vi "ep_Simulate.vi"(0 "signal definition":T2(array[cluster])=[{"Array"=[{"level (%)"=100.0, "phase (°)"=0.0, "harm."=1.0}, {"level (%)"=3.0, "phase (°)"=30.0, "harm."=3.0}]}, {"Array"=[{"level (%)"=100.0, "phase (°)"=-120.0, "harm."=1.0}, {"level (%)"=4.0, "phase (°)"=80.0, "harm."=7.0}]}, {"Array"=[{"level (%)"=100.0, "phase (°)"=-240.0, "harm."=1.0}, {"level (%)"=2.0, "phase (°)"=140.0, "harm."=5.0}]}, {"Array"=[{"level (%)"=100.0, "phase (°)"=10.0, "harm."=1.0}, {"level (%)"=6.0, "phase (°)"=0.0, "harm."=2.0}]}, {"Array"=[{"level (%)"=100.0, "phase (°)"=-105.0, "harm."=1.0}, {"level (%)"=2.0, "phase (°)"=0.0, "harm."=13.0}]}, {"Array"=[{"level (%)"=100.0, "phase (°)"=-235.0, "harm."=1.0}, {"level (%)"=4.0, "phase (°)"=60.0, "harm."=15.0}]}, {"Array"=[{"level (%)"=20.0, "phase (°)"=35.0, "harm."=1.0}, {"level (%)"=1.0, "phase (°)"=200.0, "harm."=7.0}]}], 1 "AI data channel order":T3[](array[typedef])=[enum."Voltage Phase A (L1)", enum."Voltage Phase B (L2)", enum."Voltage Phase C (L3)", enum."Current Phase A (L1)", enum."Current Phase B (L2)", enum."Current Phase C (L3)", enum."Current Phase N (Neutral)"], 9 "system info in":refnum<class "EP System Info.lvclass">=refnum, 11 "error in (no error)":errorcluster) -> (4 "AI data":sgl[][](array[numeric]) format="%#.21g", 6 "sampling rate (Hz)":sgl=9600.0 format="%#.6g", 8 "RT controler time":timestamp=timestamp(3405305275.2054996 s since 1904-01-01), 10 "system info out":refnum<class "EP System Info.lvclass">, 14 "DI data":u16[][](array[numeric])=[[0, 0], [0, 0], [0, 0], [0, 0], [0, 0], [0, 0], [0, 0], [0, 0], [0, 0], [0, 0], [0, 0], [0, 0], [0, 0], [0, 0], [0, 0], [0, 0], [0, 0], [0, 0], [0, 0], [0, 0], [0, 0], [0, 0], [0, 0], [0, 0], [0, 0], [0, 0], [0, 0], [0, 0], [0, 0], [0, 0], [3, 0], [3, 0], [3, 0], [3, 0], [3, 0], [3, 0], [3, 0], [3, 0], [3, 0], [3, 0], [3, 0], [3, 0], [3, 0], [3, 0], [3, 0], [3, 0], [3, 0], [3, 0], [3, 0], [3, 0], [0, 0], [0, 0], [0, 0], [0, 0], [0, 0], [0, 0], [0, 0], [0, 0], [0, 0], [0, 0], [0, 3], [0, 3], [0, 3], [0, 3], [0, 3], [0, 3], [0, 3], [0, 3], [0, 3], [0, 3], [0, 3], [0, 3], [0, 3], [0, 3], [0, 3], [0, 3], [0, 3], [0, 3], [0, 3], [0, 3], [0, 3], [0, 3], [0, 3], [0, 3], [0, 3], [0, 3], [0, 3], [0, 3], [0, 3], [0, 3], [0, 0], [0, 0], [0, 0], [0, 0], [0, 0], [0, 0], [0, 0], [0, 0], [0, 0], [0, 0], [0, 0], [0, 0], [0, 0], [0, 0], [0, 0], [0, 0], [0, 0], [0, 0], [0, 0], [0, 0], [0, 0], [0, 0], [0, 0], [0, 0], [0, 0], [0, 0], [0, 0], [0, 0], [0, 0], [0, 0], [0, 0], [0, 0], [0, 0], [0, 0], [0, 0], [0, 0], [0, 0], [0, 0], [0, 0], [0, 0], [0, 0], [0, 0], [0, 0], [0, 0], [0, 0], [0, 0], [0, 0], [0, 0], [0, 0], [0, 0], [0, 0], [0, 0], [0, 0], [0, 0], [0, 0], [0, 0], [0, 0], [0, 0], [0, 0], [0, 0], [0, 0], [0, 0], [0, 0], [0, 0], [0, 0], [0, 0], [0, 0], [0, 0], [0, 0], [0, 0], [0, 0], [0, 0], [0, 0], [0, 0], [0, 0], [0, 0], [0, 0], [0, 0], [0, 0], [0, 0], [0, 0], [0, 0], [0, 0], [0, 0], [0, 0], [0, 0], [0, 0], [0, 0], [0, 0], [0, 0], [0, 0], [0, 0], [0, 0], [0, 0], [0, 0], [0, 0], [0, 0], [0, 0], [0, 0], [0, 0], [0, 0], [0, 0], [0, 0], [0, 0], [0, 0], [0, 0], [0, 0], [0, 0], [0, 0], [0, 0], [0, 0], [0, 0], [0, 0], [0, 0], [0, 0], [0, 0], [0, 0], [0, 0], [0, 0], [0, 0], [0, 0], [0, 0], [0, 0], [0, 0], [0, 0], [0, 0], [0, 0], [0, 0], [0, 0], [0, 0], [0, 0], [0, 0], [0, 0], [0, 0], [0, 0], [0, 0], [0, 0], [0, 0], [0, 0], [0, 0], [0, 0], [0, 0], [0, 0], [0, 0], [0, 0], [0, 0], [0, 0], [0, 0], [0, 0], [0, 0], [0, 0], [0, 0], [0, 0], [0, 0], [0, 0], [0, 0], [0, 0], [0, 0], [0, 0], [0, 0], [0, 0], [0, 0], [0, 0], [0, 0], [0, 0], [0, 0], [0, 0], [0, 0], [0, 0], [0, 0], [0, 0], [0, 0], [0, 0], [0, 0], [0, 0], [0, 0], [0, 0], [0, 0], [0, 0], [0, 0], [0, 0], [0, 0], [0, 0], [0, 0], [0, 0], [0, 0], [0, 0], [0, 0], [0, 0], [0, 0], [0, 0], [0, 0], [0, 0], [0, 0], [0, 0], [0, 0], [0, 0], [0, 0], [0, 0], [0, 0], [0, 0], [0, 0], [0, 0], [0, 0], [0, 0], [0, 0], [0, 0], [0, 0], [0, 0], [0, 0], [0, 0], [0, 0], [0, 0], [0, 0], [0, 0], [0, 0], [0, 0], [0, 0], [0, 0], [0, 0], [0, 0], [0, 0], [0, 0], [0, 0], [0, 0], [0, 0], [0, 0], [0, 0], [0, 0], [0, 0], [0, 0], [0, 0], [0, 0], [0, 0], [0, 0], [0, 0], [0, 0], [0, 0], [0, 0], [0, 0], [0, 0], [0, 0], [0, 0], [0, 0], [0, 0], [0, 0], [0, 0], [0, 0], [0, 0], [0, 0], [0, 0], [0, 0], [0, 0], [0, 0], [0, 0], [0, 0], [0, 0], [0, 0], [0, 0], [0, 0], [0, 0], [0, 0], [0, 0], [0, 0], [0, 0], [0, 0], [0, 0], [0, 0], [0, 0], [0, 0], [0, 0], [0, 0], [0, 0], [0, 0], [0, 0], [0, 0], [0, 0], [0, 0], [0, 0], [0, 0], [0, 0], [0, 0], [0, 0], [0, 0], [0, 0], [0, 0], [0, 0], [0, 0], [0, 0], [0, 0], [0, 0], [0, 0], [0, 0], [0, 0], [0, 0], [0, 0], [0, 0], [0, 0], [0, 0], [0, 0], [0, 0], [0, 0], [0, 0], [0, 0], [0, 0], [0, 0], [0, 0], [0, 0], [0, 0], [0, 0], [0, 0], [0, 0], [0, 0], [0, 0], [0, 0], [0, 0], [0, 0], [0, 0], [0, 0], [0, 0], [0, 0], [0, 0], [0, 0], [0, 0], [0, 0], [0, 0], [0, 0], [0, 0], [0, 0], [0, 0], [0, 0], [0, 0], [0, 0], [0, 0], [0, 0], [0, 0], [0, 0], [0, 0], [0, 0], [0, 0], [0, 0], [0, 0], [0, 0], [0, 0], [0, 0], [0, 0], [0, 0], [0, 0], [0, 0], [0, 0], [0, 0], [0, 0], [0, 0], [0, 0], [0, 0], [0, 0], [0, 0], [0, 0], [0, 0], [0, 0], [0, 0], [0, 0], [0, 0], [0, 0], [0, 0], [0, 0], [0, 0], [0, 0], [0, 0], [0, 0], [0, 0], [0, 0], [0, 0], [0, 0], [0, 0], [0, 0], [0, 0], [0, 0], [0, 0], [0, 0], [0, 0], [0, 0], [0, 0], [0, 0], [0, 0], [0, 0], [0, 0], [0, 0], [0, 0], [0, 0], [0, 0], [0, 0], [0, 0], [0, 0], [0, 0], [0, 0], [0, 0], [0, 0], [0, 0], [0, 0], [0, 0], [0, 0], [0, 0], [0, 0], [0, 0], [0, 0], [0, 0], [0, 0], [0, 0], [0, 0], [0, 0], [0, 0], [0, 0], [0, 0], [0, 0], [0, 0], [0, 0], [0, 0], [0, 0], [0, 0], [0, 0], [0, 0], [0, 0], [0, 0], [0, 0], [0, 0], [0, 0], [0, 0], [0, 0], [0, 0], [0, 0], [0, 0], [0, 0], [0, 0], [0, 0], [0, 0], [0, 0], [0, 0], [0, 0], [0, 0], [0, 0], [0, 0], [0, 0], [0, 0], [0, 0], [0, 0], [0, 0], [0, 0], [0, 0], [0, 0], [0, 0], [0, 0], [0, 0], [0, 0], [0, 0], [0, 0], [0, 0], [0, 0], [0, 0], [0, 0], [0, 0], [0, 0], [0, 0], [0, 0], [0, 0], [0, 0], [0, 0], [0, 0], [0, 0], [0, 0], [0, 0], [0, 0], [0, 0], [0, 0], [0, 0], [0, 0], [0, 0], [0, 0], [0, 0], [0, 0], [0, 0], [0, 0], [0, 0], [0, 0], [0, 0], [0, 0], [0, 0], [0, 0], [0, 0], [0, 0], [0, 0], [0, 0], [0, 0], [0, 0], [0, 0], [0, 0], [0, 0], [0, 0], [0, 0], [0, 0], [0, 0], [0, 0], [0, 0], [0, 0], [0, 0], [0, 0], [0, 0], [0, 0], [0, 0], [0, 0], [0, 0], [0, 0], [0, 0], [0, 0], [0, 0], [0, 0], [0, 0], [0, 0], [0, 0], [0, 0], [0, 0], [0, 0], [0, 0], [0, 0], [0, 0], [0, 0], [0, 0], [0, 0], [0, 0], [0, 0], [0, 0], [0, 0], [0, 0], [0, 0], [0, 0], [0, 0], [0, 0], [0, 0], [0, 0], [0, 0], [0, 0], [0, 0], [0, 0], [0, 0], [0, 0], [0, 0], [0, 0], [0, 0], [0, 0], [0, 0], [0, 0], [0, 0], [0, 0], [0, 0], [0, 0], [0, 0], [0, 0], [0, 0], [0, 0], [0, 0], [0, 0], [0, 0], [0, 0], [0, 0], [0, 0], [0, 0], [0, 0], [0, 0], [0, 0], [0, 0], [0, 0], [0, 0], [0, 0], [0, 0], [0, 0], [0, 0], [0, 0], [0, 0], [0, 0], [0, 0], [0, 0], [0, 0], [0, 0], [0, 0], [0, 0], [0, 0], [0, 0], [0, 0], [0, 0], [0, 0], [0, 0], [0, 0], [0, 0], [0, 0], [0, 0], [0, 0], [0, 0], [0, 0], [0, 0], [0, 0], [0, 0], [0, 0], [0, 0], [0, 0], [0, 0], [0, 0], [0, 0], [0, 0], [0, 0], [0, 0], [0, 0], [0, 0], [0, 0], [0, 0], [0, 0], [0, 0], [0, 0], [0, 0], [0, 0], [0, 0], [0, 0], [0, 0], [0, 0], [0, 0], [0, 0], [0, 0], [0, 0], [0, 0], [0, 0], [0, 0], [0, 0], [0, 0], [0, 0], [0, 0], [0, 0], [0, 0], [0, 0], [0, 0], [0, 0], [0, 0], [0, 0], [0, 0], [0, 0], [0, 0], [0, 0], [0, 0], [0, 0], [0, 0], [0, 0], [0, 0], [0, 0], [0, 0], [0, 0], [0, 0], [0, 0], [0, 0], [0, 0], [0, 0], [0, 0], [0, 0], [0, 0], [0, 0], [0, 0], [0, 0], [0, 0], [0, 0], [0, 0], [0, 0], [0, 0], [0, 0], [0, 0], [0, 0], [0, 0], [0, 0], [0, 0], [0, 0], [0, 0], [0, 0], [0, 0], [0, 0], [0, 0], [0, 0], [0, 0], [0, 0], [0, 0], [0, 0], [0, 0], [0, 0], [0, 0], [0, 0], [0, 0], [0, 0], [0, 0], [0, 0], [0, 0], [0, 0], [0, 0], [0, 0], [0, 0], [0, 0], [0, 0], [0, 0], [0, 0], [0, 0], [0, 0], [0, 0], [0, 0], [0, 0], [0, 0], [0, 0], [0, 0], [0, 0], [0, 0], [0, 0], [0, 0], [0, 0], [0, 0], [0, 0], [0, 0], [0, 0], [0, 0], [0, 0], [0, 0], [0, 0], [0, 0], [0, 0], [0, 0], [0, 0], [0, 0], [0, 0], [0, 0], [0, 0], [0, 0], [0, 0], [0, 0], [0, 0], [0, 0], [0, 0], [0, 0], [0, 0], [0, 0], [0, 0], [0, 0], [0, 0], [0, 0], [0, 0], [0, 0], [0, 0], [0, 0], [0, 0], [0, 0], [0, 0], [0, 0], [0, 0], [0, 0], [0, 0], [0, 0], [0, 0], [0, 0], [0, 0], [0, 0], [0, 0], [0, 0], [0, 0], [0, 0], [0, 0], [0, 0], [0, 0], [0, 0], [0, 0], [0, 0], [0, 0], [0, 0], [0, 0], [0, 0], [0, 0], [0, 0], [0, 0], [0, 0], [0, 0], [0, 0], [0, 0], [0, 0], [0, 0], [0, 0], [0, 0], [0, 0], [0, 0], [0, 0], [0, 0], [0, 0], [0, 0], [0, 0], [0, 0], [0, 0], [0, 0], [0, 0], [0, 0], [0, 0], [0, 0], [0, 0], [0, 0], [0, 0], [0, 0], [0, 0], [0, 0], [0, 0], [0, 0], [0, 0], [0, 0], [0, 0], [0, 0], [0, 0], [0, 0], [0, 0], [0, 0], [0, 0], [0, 0], [0, 0], [0, 0], [0, 0], [0, 0], [0, 0], [0, 0], [0, 0], [0, 0], [0, 0], [0, 0], [0, 0], [0, 0], [0, 0], [0, 0], [0, 0], [0, 0], [0, 0], [0, 0], [0, 0], [0, 0], [0, 0], [0, 0], [0, 0], [0, 0], [0, 0], [0, 0], [0, 0], [0, 0], [0, 0], [0, 0], [0, 0], [0, 0], [0, 0], [0, 0], [0, 0], [0, 0], [0, 0], [0, 0], [0, 0], [0, 0], [0, 0], [0, 0], [0, 0], [0, 0], [0, 0], [0, 0], [0, 0], [0, 0], [0, 0], [0, 0], [0, 0], [0, 0], [0, 0], [0, 0], [0, 0], [0, 0], [0, 0], [0, 0], [0, 0], [0, 0], [0, 0], [0, 0], [0, 0], [0, 0], [0, 0], [0, 0], [0, 0], [0, 0], [0, 0], [0, 0], [0, 0], [0, 0], [0, 0], [0, 0], [0, 0], [0, 0], [0, 0], [0, 0], [0, 0], [0, 0], [0, 0], [0, 0], [0, 0], [0, 0], [0, 0], [0, 0], [0, 0], [0, 0], [0, 0], [0, 0], [0, 0], [0, 0], [0, 0], [0, 0], [0, 0], [0, 0], [0, 0], [0, 0], [0, 0], [0, 0], [0, 0], [0, 0], [0, 0], [0, 0], [0, 0], [0, 0], [0, 0], [0, 0], [0, 0], [0, 0], [0, 0], [0, 0], [0, 0], [0, 0], [0, 0], [0, 0], [0, 0], [0, 0], [0, 0], [0, 0], [0, 0], [0, 0], [0, 0], [0, 0], [0, 0], [0, 0], [0, 0], [0, 0], [0, 0], [0, 0], [0, 0], [0, 0], [0, 0], [0, 0], [0, 0], [0, 0], [0, 0], [0, 0], [0, 0], [0, 0], [0, 0], [0, 0], [0, 0], [0, 0], [0, 0], [0, 0], [0, 0], [0, 0], [0, 0], [0, 0], [0, 0], [0, 0], [0, 0], [0, 0], [0, 0], [0, 0], [0, 0], [0, 0], [0, 0], [0, 0], [0, 0], [0, 0], [0, 0], [0, 0], [0, 0], [0, 0], [0, 0], [0, 0], [0, 0], [0, 0], [0, 0], [0, 0], [0, 0], [0, 0], [0, 0], [0, 0], [0, 0], [0, 0], [0, 0], [0, 0], [0, 0], [0, 0], [0, 0], [0, 0], [0, 0], [0, 0], [0, 0], [0, 0], [0, 0], [0, 0], [0, 0], [0, 0], [0, 0], [0, 0], [0, 0], [0, 0], [0, 0], [0, 0], [0, 0], [0, 0], [0, 0], [0, 0], [0, 0], [0, 0], [0, 0], [0, 0], [0, 0], [0, 0], [0, 0], [0, 0], [0, 0], [0, 0], [0, 0], [0, 0], [0, 0], [0, 0], [0, 0], [0, 0], [0, 0], [0, 0], [0, 0], [0, 0], [0, 0], [0, 0], [0, 0], [0, 0], [0, 0], [0, 0], [0, 0], [0, 0], [0, 0], [0, 0], [0, 0], [0, 0], [0, 0], [0, 0], [0, 0], [0, 0], [0, 0], [0, 0], [0, 0], [0, 0], [0, 0], [0, 0], [0, 0], [0, 0], [0, 0], [0, 0], [0, 0], [0, 0], [0, 0], [0, 0], [0, 0], [0, 0], [0, 0], [0, 0], [0, 0], [0, 0], [0, 0], [0, 0], [0, 0], [0, 0], [0, 0], [0, 0], [0, 0], [0, 0], [0, 0], [0, 0], [0, 0], [0, 0], [0, 0], [0, 0], [0, 0], [0, 0], [0, 0], [0, 0], [0, 0], [0, 0], [0, 0], [0, 0], [0, 0], [0, 0], [0, 0], [0, 0], [0, 0], [0, 0], [0, 0], [0, 0], [0, 0], [0, 0], [0, 0], [0, 0], [0, 0], [0, 0], [0, 0], [0, 0], [0, 0], [0, 0], [0, 0], [0, 0], [0, 0], [0, 0], [0, 0], [0, 0], [0, 0], [0, 0], [0, 0], [0, 0], [0, 0], [0, 0], [0, 0], [0, 0], [0, 0], [0, 0], [0, 0], [0, 0], [0, 0], [0, 0], [0, 0], [0, 0], [0, 0], [0, 0], [0, 0], [0, 0], [0, 0], [0, 0], [0, 0], [0, 0], [0, 0], [0, 0], [0, 0], [0, 0], [0, 0], [0, 0], [0, 0], [0, 0], [0, 0], [0, 0], [0, 0], [0, 0], [0, 0], [0, 0], [0, 0], [0, 0], [0, 0], [0, 0], [0, 0], [0, 0], [0, 0], [0, 0], [0, 0], [0, 0], [0, 0], [0, 0], [0, 0], [0, 0], [0, 0], [0, 0], [0, 0], [0, 0], [0, 0], [0, 0], [0, 0], [0, 0], [0, 0], [0, 0], [0, 0], [0, 0], [0, 0], [0, 0], [0, 0], [0, 0], [0, 0], [0, 0], [0, 0], [0, 0], [0, 0], [0, 0], [0, 0], [0, 0], [0, 0], [0, 0], [0, 0], [0, 0], [0, 0], [0, 0], [0, 0], [0, 0], [0, 0], [0, 0], [0, 0], [0, 0], [0, 0], [0, 0], [0, 0], [0, 0], [0, 0], [0, 0], [0, 0], [0, 0], [0, 0], [0, 0], [0, 0], [0, 0], [0, 0], [0, 0], [0, 0], [0, 0], [0, 0], [0, 0], [0, 0], [0, 0], [0, 0], [0, 0], [0, 0], [0, 0], [0, 0], [0, 0], [0, 0], [0, 0], [0, 0], [0, 0], [0, 0], [0, 0], [0, 0], [0, 0], [0, 0], [0, 0], [0, 0], [0, 0], [0, 0], [0, 0], [0, 0], [0, 0], [0, 0], [0, 0], [0, 0], [0, 0], [0, 0], [0, 0], [0, 0], [0, 0], [0, 0], [0, 0], [0, 0], [0, 0], [0, 0], [0, 0], [0, 0], [0, 0], [0, 0], [0, 0], [0, 0], [0, 0], [0, 0], [0, 0], [0, 0], [0, 0], [0, 0], [0, 0], [0, 0], [0, 0], [0, 0], [0, 0], [0, 0], [0, 0], [0, 0], [0, 0], [0, 0], [0, 0], [0, 0], [0, 0], [0, 0], [0, 0], [0, 0], [0, 0], [0, 0], [0, 0], [0, 0], [0, 0], [0, 0], [0, 0], [0, 0], [0, 0], [0, 0], [0, 0], [0, 0], [0, 0], [0, 0], [0, 0], [0, 0], [0, 0], [0, 0], [0, 0], [0, 0], [0, 0], [0, 0], [0, 0], [0, 0], [0, 0], [0, 0], [0, 0], [0, 0], [0, 0], [0, 0], [0, 0], [0, 0], [0, 0], [0, 0], [0, 0], [0, 0], [0, 0], [0, 0], [0, 0], [0, 0], [0, 0], [0, 0], [0, 0], [0, 0], [0, 0], [0, 0], [0, 0], [0, 0], [0, 0], [0, 0], [0, 0], [0, 0], [0, 0], [0, 0], [0, 0], [0, 0], [0, 0], [0, 0], [0, 0], [0, 0], [0, 0], [0, 0], [0, 0], [0, 0], [0, 0], [0, 0], [0, 0], [0, 0], [0, 0], [0, 0], [0, 0], [0, 0], [0, 0], [0, 0], [0, 0], [0, 0], [0, 0], [0, 0], [0, 0], [0, 0], [0, 0], [0, 0], [0, 0], [0, 0], [0, 0], [0, 0], [0, 0], [0, 0], [0, 0], [0, 0], [0, 0], [0, 0], [0, 0], [0, 0], [0, 0], [0, 0], [0, 0], [0, 0], [0, 0], [0, 0], [0, 0], [0, 0], [0, 0], [0, 0], [0, 0], [0, 0], [0, 0], [0, 0], [0, 0], [0, 0], [0, 0], [0, 0], [0, 0], [0, 0], [0, 0], [0, 0], [0, 0], [0, 0], [0, 0], [0, 0], [0, 0], [0, 0], [0, 0], [0, 0], [0, 0], [0, 0], [0, 0], [0, 0], [0, 0], [0, 0], [0, 0], [0, 0], [0, 0], [0, 0], [0, 0], [0, 0], [0, 0], [0, 0], [0, 0], [0, 0], [0, 0], [0, 0], [0, 0], [0, 0], [0, 0], [0, 0], [0, 0], [0, 0], [0, 0], [0, 0], [0, 0], [0, 0], [0, 0], [0, 0], [0, 0], [0, 0], [0, 0], [0, 0], [0, 0], [0, 0], [0, 0], [0, 0], [0, 0], [0, 0], [0, 0], [0, 0], [0, 0], [0, 0], [0, 0], [0, 0], [0, 0], [0, 0], [0, 0], [0, 0], [0, 0], [0, 0], [0, 0], [0, 0], [0, 0], [0, 0], [0, 0], [0, 0], [0, 0], [0, 0], [0, 0], [0, 0], [0, 0], [0, 0], [0, 0], [0, 0], [0, 0], [0, 0], [0, 0], [0, 0], [0, 0], [0, 0], [0, 0], [0, 0], [0, 0], [0, 0], [0, 0], [0, 0], [0, 0], [0, 0], [0, 0], [0, 0], [0, 0], [0, 0], [0, 0], [0, 0], [0, 0], [0, 0], [0, 0], [0, 0], [0, 0], [0, 0], [0, 0], [0, 0], [0, 0], [0, 0], [0, 0], [0, 0], [0, 0], [0, 0], [0, 0], [0, 0], [0, 0], [0, 0], [0, 0], [0, 0], [0, 0], [0, 0], [0, 0], [0, 0], [0, 0], [0, 0], [0, 0], [0, 0], [0, 0], [0, 0], [0, 0], [0, 0], [0, 0], [0, 0], [0, 0], [0, 0], [0, 0], [0, 0], [0, 0], [0, 0], [0, 0], [0, 0], [0, 0], [0, 0], [0, 0], [0, 0], [0, 0], [0, 0], [0, 0], [0, 0], [0, 0], [0, 0], [0, 0], [0, 0], [0, 0], [0, 0], [0, 0], [0, 0], [0, 0], [0, 0], [0, 0], [0, 0], [0, 0], [0, 0], [0, 0], [0, 0], [0, 0], [0, 0], [0, 0], [0, 0], [0, 0], [0, 0], [0, 0], [0, 0], [0, 0], [0, 0], [0, 0], [0, 0], [0, 0], [0, 0], [0, 0], [0, 0], [0, 0], [0, 0], [0, 0], [0, 0], [0, 0], [0, 0], [0, 0], [0, 0], [0, 0], [0, 0], [0, 0], [0, 0], [0, 0], [0, 0], [0, 0], [0, 0], [0, 0], [0, 0], [0, 0], [0, 0], [0, 0], [0, 0], [0, 0], [0, 0], [0, 0], [0, 0], [0, 0], [0, 0], [0, 0], [0, 0], [0, 0], [0, 0], [0, 0], [0, 0], [0, 0], [0, 0], [0, 0], [0, 0], [0, 0], [0, 0], [0, 0], [0, 0], [0, 0], [0, 0], [0, 0], [0, 0], [0, 0], [0, 0], [0, 0], [0, 0], [0, 0], [0, 0], [0, 0], [0, 0], [0, 0], [0, 0], [0, 0], [0, 0], [0, 0], [0, 0], [0, 0], [0, 0], [0, 0], [0, 0], [0, 0], [0, 0], [0, 0], [0, 0], [0, 0], [0, 0], [0, 0], [0, 0], [0, 0], [0, 0], [0, 0], [0, 0], [0, 0], [0, 0], [0, 0], [0, 0], [0, 0], [0, 0], [0, 0], [0, 0], [0, 0], [0, 0], [0, 0], [0, 0], [0, 0], [0, 0], [0, 0], [0, 0], [0, 0], [0, 0], [0, 0], [0, 0], [0, 0], [0, 0], [0, 0], [0, 0], [0, 0], [0, 0], [0, 0], [0, 0], [0, 0], [0, 0], [0, 0], [0, 0], [0, 0], [0, 0], [0, 0], [0, 0], [0, 0], [0, 0], [0, 0], [0, 0], [0, 0], [0, 0], [0, 0], [0, 0], [0, 0], [0, 0], [0, 0], [0, 0], [0, 0], [0, 0], [0, 0], [0, 0], [0, 0], [0, 0], [0, 0], [0, 0], [0, 0], [0, 0], [0, 0], [0, 0], [0, 0], [0, 0], [0, 0], [0, 0], [0, 0], [0, 0], [0, 0], [0, 0], [0, 0], [0, 0], [0, 0], [0, 0], [0, 0], [0, 0], [0, 0], [0, 0], [0, 0], [0, 0], [0, 0], [0, 0], [0, 0], [0, 0], [0, 0], [0, 0], [0, 0], [0, 0], [0, 0], [0, 0], [0, 0], [0, 0], [0, 0], [0, 0], [0, 0], [0, 0], [0, 0], [0, 0], [0, 0], [0, 0], [0, 0], [0, 0], [0, 0], [0, 0], [0, 0], [0, 0], [0, 0], [0, 0], [0, 0], [0, 0], [0, 0], [0, 0], [0, 0], [0, 0], [0, 0], [0, 0], [0, 0], [0, 0], [0, 0], [0, 0], [0, 0], [0, 0], [0, 0], [0, 0], [0, 0], [0, 0], [0, 0], [0, 0], [0, 0], [0, 0], [0, 0], [0, 0], [0, 0], [0, 0], [0, 0], [0, 0], [0, 0], [0, 0], [0, 0], [0, 0], [0, 0], [0, 0], [0, 0], [0, 0], [0, 0], [0, 0], [0, 0], [0, 0], [0, 0], [0, 0], [0, 0], [0, 0], [0, 0], [0, 0], [0, 0], [0, 0], [0, 0], [0, 0], [0, 0], [0, 0], [0, 0], [0, 0], [0, 0], [0, 0], [0, 0], [0, 0], [0, 0], [0, 0], [0, 0], [0, 0], [0, 0]], 15 "error out":errorcluster)   [LabVIEW 2014]
uses:
  <vilib>/addons/Electrical Power/PQ/Common/Classes/System Info/EP System Info.lvclass
  <vilib>/addons/Electrical Power/PQ/Common/Controls/ep_AI Data Channel.ctl
  <vilib>/Analysis/NI_AALBase.lvlib
  <vilib>/addons/Electrical Power/PQ/NI_EP_Power Quality.lvlib
panel:
  out "AI data graph":sgl[][](graph)=[[4.879037, 16.326368, 27.707563, 39.004017, 50.19774, 61.271446, 72.2086, 82.99353, 93.61142, 104.04838, 114.29151, 124.32891, 134.1497, 143.744, 153.10307, 162.21907, 171.08531, 179.69598, 188.04634, 196.13255, 203.95163, 211.50146, 218.78072, 225.78876, 232.52557, 238.99178, 245.18849, 251.11716, 256.77966, 262.1781, 267.31476, 272.19202, 276.8123, 281.1779, 285.29105, 289.1538, 292.76788, 296.1347, 299.2554, 302.13052, 304.76028, 307.14435, 309.28198, 311.17178, 312.8118, 314.19968, 315.3325, 316.2067, 316.8184, 317.16315, 317.23618, 317.03232, 316.54605, 315.7717, 314.70328, 313.3348, 311.66028, 309.6736, 307.36893, 304.74057, 301.78317, 298.4917, 294.86163, 290.88898, 286.57034, 281.9031, 276.88535, 271.516, 265.79495, 259.72302, 253.30203, 246.53488, 239.42557, 231.9792, 224.20201, 216.1014, 207.68588, 198.96516, 189.95006, 180.65244, 171.08531, 161.26262, 151.19936, 140.91139, 130.41545, 119.72899, 108.87022, 97.85792, 86.71142, 75.45044, 64.09506, 52.665592, 41.182453, 29.666122, 18.13699, 6.615282, -4.879037, -16.326368, -27.707563, -39.004017, -50.19774, -61.271446, -72.2086, -82.99353, -93.61142, -104.04838, -114.29151, -124.32891, -134.1497, -143.744, -153.10307, -162.21907, -171.08531, -179.69598, -188.04634, -196.13255, -203.95163, -211.50146, -218.78072, -225.78876, -232.52557, -238.99178, -245.18849, -251.11716, -256.77966, -262.1781, -267.31476, -272.19202, -276.8123, -281.1779, -285.29105, -289.1538, -292.76788, -296.1347, -299.2554, -302.13052, -304.76028, -307.14435, -309.28198, -311.17178, -312.8118, -314.19968, -315.3325, -316.2067, -316.8184, -317.16315, -317.23618, -317.03232, -316.54605, -315.7717, -314.70328, -313.3348, -311.66028, -309.6736, -307.36893, -304.74057, -301.78317, -298.4917, -294.86163, -290.88898, -286.57034, -281.9031, -276.88535, -271.516, -265.79495, -259.72302, -253.30203, -246.53488, -239.42557, -231.9792, -224.20201, -216.1014, -207.68588, -198.96516, -189.95006, -180.65244, -171.08531, -161.26262, -151.19936, -140.91139, -130.41545, -119.72899, -108.87022, -97.85792, -86.71142, -75.45044, -64.09506, -52.665592, -41.182453, -29.666122, -18.13699, -6.615282], [-268.8782, -273.87033, -279.234, -284.93793, -290.91696, -297.07532, -303.29153, -309.4243, -315.31982, -320.81964, -325.7688, -330.0237, -333.45956, -335.97678, -337.50613, -338.01218, -337.49524, -335.99124, -333.5698, -330.33075, -326.3988, -321.91714, -317.03992, -311.9245, -306.72318, -301.5753, -296.60025, -291.89133, -287.5111, -283.4882, -279.8161, -276.45383, -273.32816, -270.33777, -267.35892, -264.25198, -260.8694, -257.06332, -252.69402, -247.63736, -241.79176, -235.08379, -227.4725, -218.95197, -209.55199, -199.337, -188.40323, -176.874, -164.89386, -152.62152, -140.22206, -127.85876, -115.68516, -103.8375, -92.42819, -81.540474, -71.22459, -61.49572, -52.333797, -43.68506, -35.46546, -27.565634, -19.857178, -12.199944, -4.4499435, 3.5325484, 11.875112, 20.685928, 30.047552, 40.012016, 50.59752, 61.78692, 73.528046, 85.735855, 98.296295, 111.07175, 123.907585, 136.63977, 149.10289, 161.13818, 172.6014, 183.36969, 193.34775, 202.472, 210.71365, 218.07962, 224.61172, 230.38405, 235.49858, 240.07956, 244.26645, 248.20628, 252.04564, 255.92255, 259.95892, 264.25388, 268.8782, 273.87033, 279.234, 284.93793, 290.91696, 297.07532, 303.29153, 309.4243, 315.31982, 320.81964, 325.7688, 330.0237, 333.45956, 335.97678, 337.50613, 338.01218, 337.49524, 335.99124, 333.5698, 330.33075, 326.3988, 321.91714, 317.03992, 311.9245, 306.72318, 301.5753, 296.60025, 291.89133, 287.5111, 283.4882, 279.8161, 276.45383, 273.32816, 270.33777, 267.35892, 264.25198, 260.8694, 257.06332, 252.69402, 247.63736, 241.79176, 235.08379, 227.4725, 218.95197, 209.55199, 199.337, 188.40323, 176.874, 164.89386, 152.62152, 140.22206, 127.85876, 115.68516, 103.8375, 92.42819, 81.540474, 71.22459, 61.49572, 52.333797, 43.68506, 35.46546, 27.565634, 19.857178, 12.199944, 4.4499435, -3.5325484, -11.875112, -20.685928, -30.047552, -40.012016, -50.59752, -61.78692, -73.528046, -85.735855, -98.296295, -111.07175, -123.907585, -136.63977, -149.10289, -161.13818, -172.6014, -183.36969, -193.34775, -202.472, -210.71365, -218.07962, -224.61172, -230.38405, -235.49858, -240.07956, -244.26645, -248.20628, -252.04564, -255.92255, -259.95892, -264.25388], [285.8729, 279.5332, 272.80917, 265.73257, 258.3371, 250.65771, 242.72989, 234.58879, 226.26866, 217.80193, 209.2186, 200.54578, 191.80699, 183.02193, 174.20601, 165.37032, 156.52151, 147.66182, 138.78941, 129.89845, 120.97977, 112.02115, 103.008095, 93.924385, 84.75282, 75.47597, 66.07687, 56.53985, 46.851112, 36.99951, 26.977062, 16.779474, 6.406551, -4.137512, -14.843949, -25.699364, -36.685795, -47.780907, -58.958298, -70.18791, -81.436554, -92.66848, -103.84611, -114.9307, -125.883125, -136.66464, -147.23767, -157.56648, -167.61798, -177.36217, -186.7729, -195.82817, -204.51048, -212.80714, -220.71033, -228.21701, -235.3289, -242.05214, -248.39697, -254.37717, -260.00955, -265.31335, -270.30948, -275.01978, -279.46634, -283.67072, -287.65314, -291.43195, -295.02292, -298.43863, -301.6882, -304.77673, -307.70523, -310.4704, -313.06473, -315.4765, -317.69012, -319.68655, -321.44366, -322.9368, -324.1395, -325.02402, -325.56232, -325.72662, -325.49023, -324.8283, -323.7184, -322.1414, -320.08173, -317.52814, -314.47385, -310.917, -306.86066, -302.31287, -297.28653, -291.79926, -285.8729, -279.5332, -272.80917, -265.73257, -258.3371, -250.65771, -242.72989, -234.58879, -226.26866, -217.80193, -209.2186, -200.54578, -191.80699, -183.02193, -174.20601, -165.37032, -156.52151, -147.66182, -138.78941, -129.89845, -120.97977, -112.02115, -103.008095, -93.924385, -84.75282, -75.47597, -66.07687, -56.53985, -46.851112, -36.99951, -26.977062, -16.779474, -6.406551, 4.137512, 14.843949, 25.699364, 36.685795, 47.780907, 58.958298, 70.18791, 81.436554, 92.66848, 103.84611, 114.9307, 125.883125, 136.66464, 147.23767, 157.56648, 167.61798, 177.36217, 186.7729, 195.82817, 204.51048, 212.80714, 220.71033, 228.21701, 235.3289, 242.05214, 248.39697, 254.37717, 260.00955, 265.31335, 270.30948, 275.01978, 279.46634, 283.67072, 287.65314, 291.43195, 295.02292, 298.43863, 301.6882, 304.77673, 307.70523, 310.4704, 313.06473, 315.4765, 317.69012, 319.68655, 321.44366, 322.9368, 324.1395, 325.02402, 325.56232, 325.72662, 325.49023, 324.8283, 323.7184, 322.1414, 320.08173, 317.52814, 314.47385, 310.917, 306.86066, 302.31287, 297.28653, 291.79926], [6.13939, 7.414064, 8.680353, 9.936458, 11.1805935, 12.410994, 13.625914, 14.823636, 16.002472, 17.160767, 18.2969, 19.409292, 20.49641, 21.556763, 22.58891, 23.591463, 24.563091, 25.502516, 26.408524, 27.279957, 28.115728, 28.914814, 29.676252, 30.399162, 31.08272, 31.726181, 32.32887, 32.89019, 33.409607, 33.88667, 34.32099, 34.71227, 35.06027, 35.364822, 35.625843, 35.843315, 36.017277, 36.147858, 36.235233, 36.279667, 36.281464, 36.241, 36.15872, 36.035114, 35.870728, 35.66617, 35.422085, 35.139187, 34.81821, 34.459953, 34.065243, 33.634937, 33.16995, 32.6712, 32.13966, 31.57631, 30.98216, 30.358238, 29.705593, 29.025288, 28.31839, 27.585987, 26.829166, 26.04902, 25.246643, 24.423134, 23.579578, 22.71707, 21.836683, 20.939495, 20.026564, 19.098946, 18.15767, 17.203762, 16.238232, 15.262067, 14.276241, 13.281707, 12.279401, 11.270241, 10.255121, 9.23492, 8.210493, 7.1826797, 6.152296, 5.1201415, 4.086996, 3.0536208, 2.0207608, 0.98914266, -0.040521502, -1.0675354, -2.0912163, -3.110895, -4.125913, -5.135624, -6.13939, -7.136582, -8.126577, -9.10876, -10.082518, -11.047241, -12.002325, -12.947164, -13.881151, -14.803681, -15.714144, -16.611925, -17.49641, -18.366978, -19.222996, -20.063837, -20.888855, -21.697409, -22.488834, -23.262474, -24.017653, -24.753693, -25.469908, -26.165604, -26.840078, -27.492622, -28.122526, -28.729069, -29.311531, -29.869184, -30.401304, -30.907162, -31.386034, -31.837196, -32.25993, -32.653526, -33.017277, -33.350487, -33.652477, -33.92258, -34.16014, -34.36453, -34.53513, -34.67136, -34.77265, -34.83847, -34.868313, -34.861706, -34.81821, -34.737434, -34.619015, -34.462635, -34.268024, -34.034954, -33.76325, -33.45278, -33.10348, -32.715324, -32.28835, -31.822655, -31.31839, -30.775772, -30.19508, -29.576647, -28.92088, -28.228241, -27.499268, -26.734552, -25.93476, -25.100613, -24.232908, -23.3325, -22.40031, -21.43732, -20.444576, -19.423187, -18.374317, -17.29919, -16.19909, -15.07535, -13.929356, -12.762546, -11.5764065, -10.372466, -9.152296, -7.9175086, -6.669752, -5.410706, -4.1420813, -2.8656147, -1.5830668, -0.2962168, 0.99314016, 2.2831967, 3.5721374, 4.858142], [28.9614, 28.574211, 28.104712, 27.510912, 26.767748, 25.871693, 24.841526, 23.715147, 22.542961, 21.379066, 20.271769, 19.255142, 18.343128, 17.527235, 16.77823, 16.051533, 15.295365, 14.460169, 13.507639, 12.417752, 11.192541, 9.855937, 8.449712, 7.0262446, 5.63939, 4.3350973, 3.1434324, 2.0734334, 1.1117189, 0.22509211, -0.63332295, -1.5155047, -2.4690485, -3.5284615, -4.7087936, -6.002733, -7.381698, -8.800709, -10.206195, -11.545334, -12.775251, -13.870458, -14.827183, -15.66385, -16.417576, -17.137363, -17.875175, -18.676464, -19.571882, -20.571646, -21.663507, -22.81479, -23.978018, -25.09921, -26.127361, -27.02335, -27.766773, -28.359434, -28.82487, -29.204016, -29.547792, -29.907879, -30.32739, -30.83308, -31.430447, -32.102673, -32.813503, -33.513645, -34.149445, -34.672398, -35.04772, -35.26048, -35.31821, -35.249523, -35.098953, -34.91899, -34.760704, -34.6646, -34.653404, -34.727997, -34.86725, -35.031815, -35.171146, -35.232544, -35.17056, -34.95515, -34.577072, -34.049595, -33.406166, -32.69453, -31.968302, -31.277449, -30.659512, -30.13297, -29.694067, -29.317574, -28.9614, -28.574211, -28.104712, -27.510912, -26.767748, -25.871693, -24.841526, -23.715147, -22.542961, -21.379066, -20.271769, -19.255142, -18.343128, -17.527235, -16.77823, -16.051533, -15.295365, -14.460169, -13.507639, -12.417752, -11.192541, -9.855937, -8.449712, -7.0262446, -5.63939, -4.3350973, -3.1434324, -2.0734334, -1.1117189, -0.22509211, 0.63332295, 1.5155047, 2.4690485, 3.5284615, 4.7087936, 6.002733, 7.381698, 8.800709, 10.206195, 11.545334, 12.775251, 13.870458, 14.827183, 15.66385, 16.417576, 17.137363, 17.875175, 18.676464, 19.571882, 20.571646, 21.663507, 22.81479, 23.978018, 25.09921, 26.127361, 27.02335, 27.766773, 28.359434, 28.82487, 29.204016, 29.547792, 29.907879, 30.32739, 30.83308, 31.430447, 32.102673, 32.813503, 33.513645, 34.149445, 34.672398, 35.04772, 35.26048, 35.31821, 35.249523, 35.098953, 34.91899, 34.760704, 34.6646, 34.653404, 34.727997, 34.86725, 35.031815, 35.171146, 35.232544, 35.17056, 34.95515, 34.577072, 34.049595, 33.406166, 32.69453, 31.968302, 31.277449, 30.659512, 30.13297, 29.694067, 29.317574], [-32.925888, -33.018295, -33.407627, -34.05936, -34.868275, -35.68325, -36.342903, -36.71368, -36.721363, -36.368595, -35.734222, -34.954723, -34.191948, -33.594955, -33.26481, -33.230797, -33.443527, -33.78668, -34.104527, -34.23881, -34.06619, -33.52747, -32.641697, -31.50176, -30.252596, -29.057085, -28.05773, -27.343145, -26.927305, -26.746391, -26.674044, -26.551394, -26.224745, -25.582094, -24.579765, -23.252937, -21.707558, -20.09554, -18.579111, -17.292747, -16.311644, -15.634208, -15.182682, -14.821766, -14.390821, -13.742075, -12.775786, -11.4640665, -9.857741, -8.07463, -6.2719936, -4.609686, -3.2126827, -2.1418586, -1.379894, -0.83566, -0.36602542, 0.19004881, 0.9731884, 2.070105, 3.4928265, 5.175569, 6.9899783, 8.775159, 10.37538, 11.676569, 12.632971, 13.277667, 13.714495, 14.093241, 14.574004, 15.289122, 16.311644, 17.637833, 19.18779, 20.824066, 22.383884, 23.717346, 24.722582, 25.36959, 25.707108, 25.850864, 25.95606, 26.18051, 26.647161, 27.4149, 28.464436, 29.702696, 30.984648, 32.147373, 33.0484, 33.599224, 33.786045, 33.672928, 33.38654, 33.08615, 32.925888, 33.018295, 33.407627, 34.05936, 34.868275, 35.68325, 36.342903, 36.71368, 36.721363, 36.368595, 35.734222, 34.954723, 34.191948, 33.594955, 33.26481, 33.230797, 33.443527, 33.78668, 34.104527, 34.23881, 34.06619, 33.52747, 32.641697, 31.50176, 30.252596, 29.057085, 28.05773, 27.343145, 26.927305, 26.746391, 26.674044, 26.551394, 26.224745, 25.582094, 24.579765, 23.252937, 21.707558, 20.09554, 18.579111, 17.292747, 16.311644, 15.634208, 15.182682, 14.821766, 14.390821, 13.742075, 12.775786, 11.4640665, 9.857741, 8.07463, 6.2719936, 4.609686, 3.2126827, 2.1418586, 1.379894, 0.83566, 0.36602542, -0.19004881, -0.9731884, -2.070105, -3.4928265, -5.175569, -6.9899783, -8.775159, -10.37538, -11.676569, -12.632971, -13.277667, -13.714495, -14.093241, -14.574004, -15.289122, -16.311644, -17.637833, -19.18779, -20.824066, -22.383884, -23.717346, -24.722582, -25.36959, -25.707108, -25.850864, -25.95606, -26.18051, -26.647161, -27.4149, -28.464436, -29.702696, -30.984648, -32.147373, -33.0484, -33.599224, -33.786045, -33.672928, -33.38654, -33.08615], [3.9348757, 4.049939, 4.170553, 4.299771, 4.4399543, 4.592639, 4.7584457, 4.93704, 5.127138, 5.326567, 5.532369, 5.7409496, 5.948256, 6.1499825, 6.341787, 6.519513, 6.6794014, 6.818277, 6.9337125, 7.024148, 7.08897, 7.1285367, 7.1441565, 7.1380153, 7.113061, 7.0728426, 7.021327, 6.962688, 6.901085, 6.8404465, 6.7842636, 6.735408, 6.695978, 6.6671968, 6.6493425, 6.641738, 6.6427884, 6.650065, 6.660436, 6.6702332, 6.6754446, 6.6719303, 6.6556435, 6.6228433, 6.5702977, 6.4954567, 6.3965917, 6.2728915, 6.1245112, 5.9525704, 5.759103, 5.5469565, 5.3196535, 5.0812135, 4.835952, 4.588264, 4.342405, 4.102273, 3.8712208, 3.651886, 3.4460652, 3.2546299, 3.0774927, 2.913621, 2.7611027, 2.6172578, 2.4787893, 2.3419669, 2.2028341, 2.0574262, 1.9019904, 1.7331929, 1.5483062, 1.3453636, 1.1232743, 0.8818934, 0.62204134, 0.34547436, 0.05480501, -0.24662173, -0.5548903, -0.86570644, -1.1746093, -1.4771913, -1.7693164, -2.0473232, -2.3082044, -2.549751, -2.7706556, -2.9705691, -3.1501062, -3.310802, -3.4550197, -3.5858166, -3.7067711, -3.8217866, -3.9348757, -4.049939, -4.170553, -4.299771, -4.4399543, -4.592639, -4.7584457, -4.93704, -5.127138, -5.326567, -5.532369, -5.7409496, -5.948256, -6.1499825, -6.341787, -6.519513, -6.6794014, -6.818277, -6.9337125, -7.024148, -7.08897, -7.1285367, -7.1441565, -7.1380153, -7.113061, -7.0728426, -7.021327, -6.962688, -6.901085, -6.8404465, -6.7842636, -6.735408, -6.695978, -6.6671968, -6.6493425, -6.641738, -6.6427884, -6.650065, -6.660436, -6.6702332, -6.6754446, -6.6719303, -6.6556435, -6.6228433, -6.5702977, -6.4954567, -6.3965917, -6.2728915, -6.1245112, -5.9525704, -5.759103, -5.5469565, -5.3196535, -5.0812135, -4.835952, -4.588264, -4.342405, -4.102273, -3.8712208, -3.651886, -3.4460652, -3.2546299, -3.0774927, -2.913621, -2.7611027, -2.6172578, -2.4787893, -2.3419669, -2.2028341, -2.0574262, -1.9019904, -1.7331929, -1.5483062, -1.3453636, -1.1232743, -0.8818934, -0.62204134, -0.34547436, -0.05480501, 0.24662173, 0.5548903, 0.86570644, 1.1746093, 1.4771913, 1.7693164, 2.0473232, 2.3082044, 2.549751, 2.7706556, 2.9705691, 3.1501062, 3.310802, 3.4550197, 3.5858166, 3.7067711, 3.8217866]]
  in  "simulate flicker":bool
  in  "fluctuations shape":enum16{"sinusoidal", "rectangular"}(ring)=enum."rectangular"
  in  "flicker frequency [Hz]":dbl=13.5
  in  "voltage fluctuation dV/V [%]":dbl=0.402
  in  "fluctuation level [%]":sgl=1.0
  in  "fluctuate signal":bool
  out "state":bool
  in  "sig eve":bool
  in  "signaling freq.":dbl=216.66
  in  "signaling voltage event settings":T1={"signaling detection threshold [%]"=0.3, "signaling starting log. 1 length (T1) [sec]"=2.99, "signaling starting log. 0 length (T2) [sec]"=2.33, "signaling message max. length [sec]"=32.0}
  in  "init":bool
  in  "current (A)":dbl(knob)=25.0 scale=0.0..50.0
  in  "voltage (V)":dbl(knob)=230.0 scale=0.0..300.0
  in  "frequency (Hz)":sgl(knob)=50.0 scale=40.0..60.0
  # "Simulated Signal Generation"
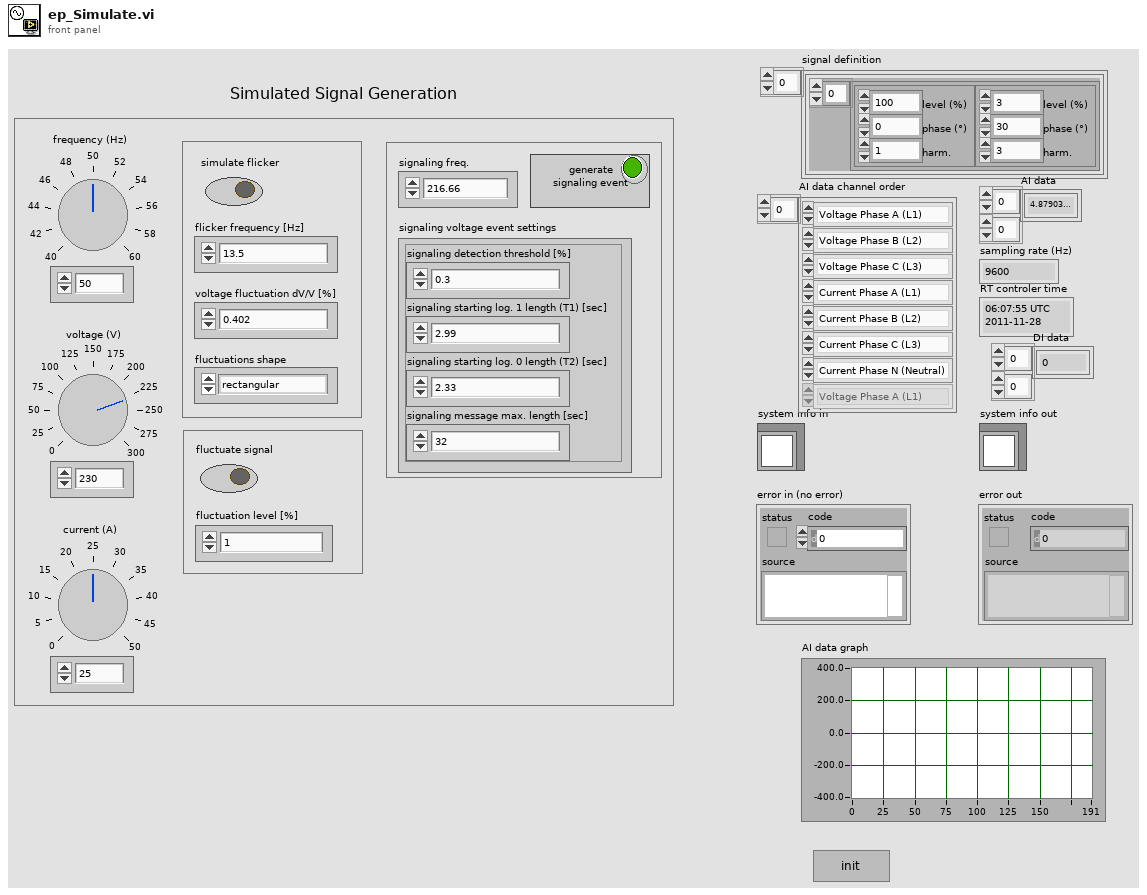
[diagram p1: front panel]
types:
  T1 = cluster{"signaling detection threshold [%]":dbl, "signaling starting log. 1 length (T1) [sec]":dbl, "signaling starting log. 0 length (T2) [sec]":dbl, "signaling message max. length [sec]":dbl}
  T2 = cluster{"Array":cluster{"level (%)":dbl, "phase (°)":dbl, "harm.":dbl}[]}[]
  T3 = typedef "NI_EP_Power Quality.lvlib/ep_AI Data Channel.ctl" = enum16{"Voltage Phase A (L1)", "Voltage Phase B (L2)", "Voltage Phase C (L3)", "Voltage Phase N (Neutral)", "Current Phase A (L1)", "Current Phase B (L2)", "Current Phase C (L3)", "Current Phase N (Neutral)"}
  T4 = enum8{"Enabled", "Disabled", "Disabled and Grayed Out"}
  T5 = typedef "NI_EP_Power Quality.lvlib/ep_Wiring.ctl" = enum16{"4xUph + 4xI", "3xUph + 4xI", "3xUline + 4xI", "3xUph + 3xI", "3xUline + 3xI", "3xUph + 2xI", "3xUline + 2xI", "1xUph + 1xI"}
  T6 = cluster{"level (%)":dbl, "phase (°)":dbl, "harm.":dbl}[]
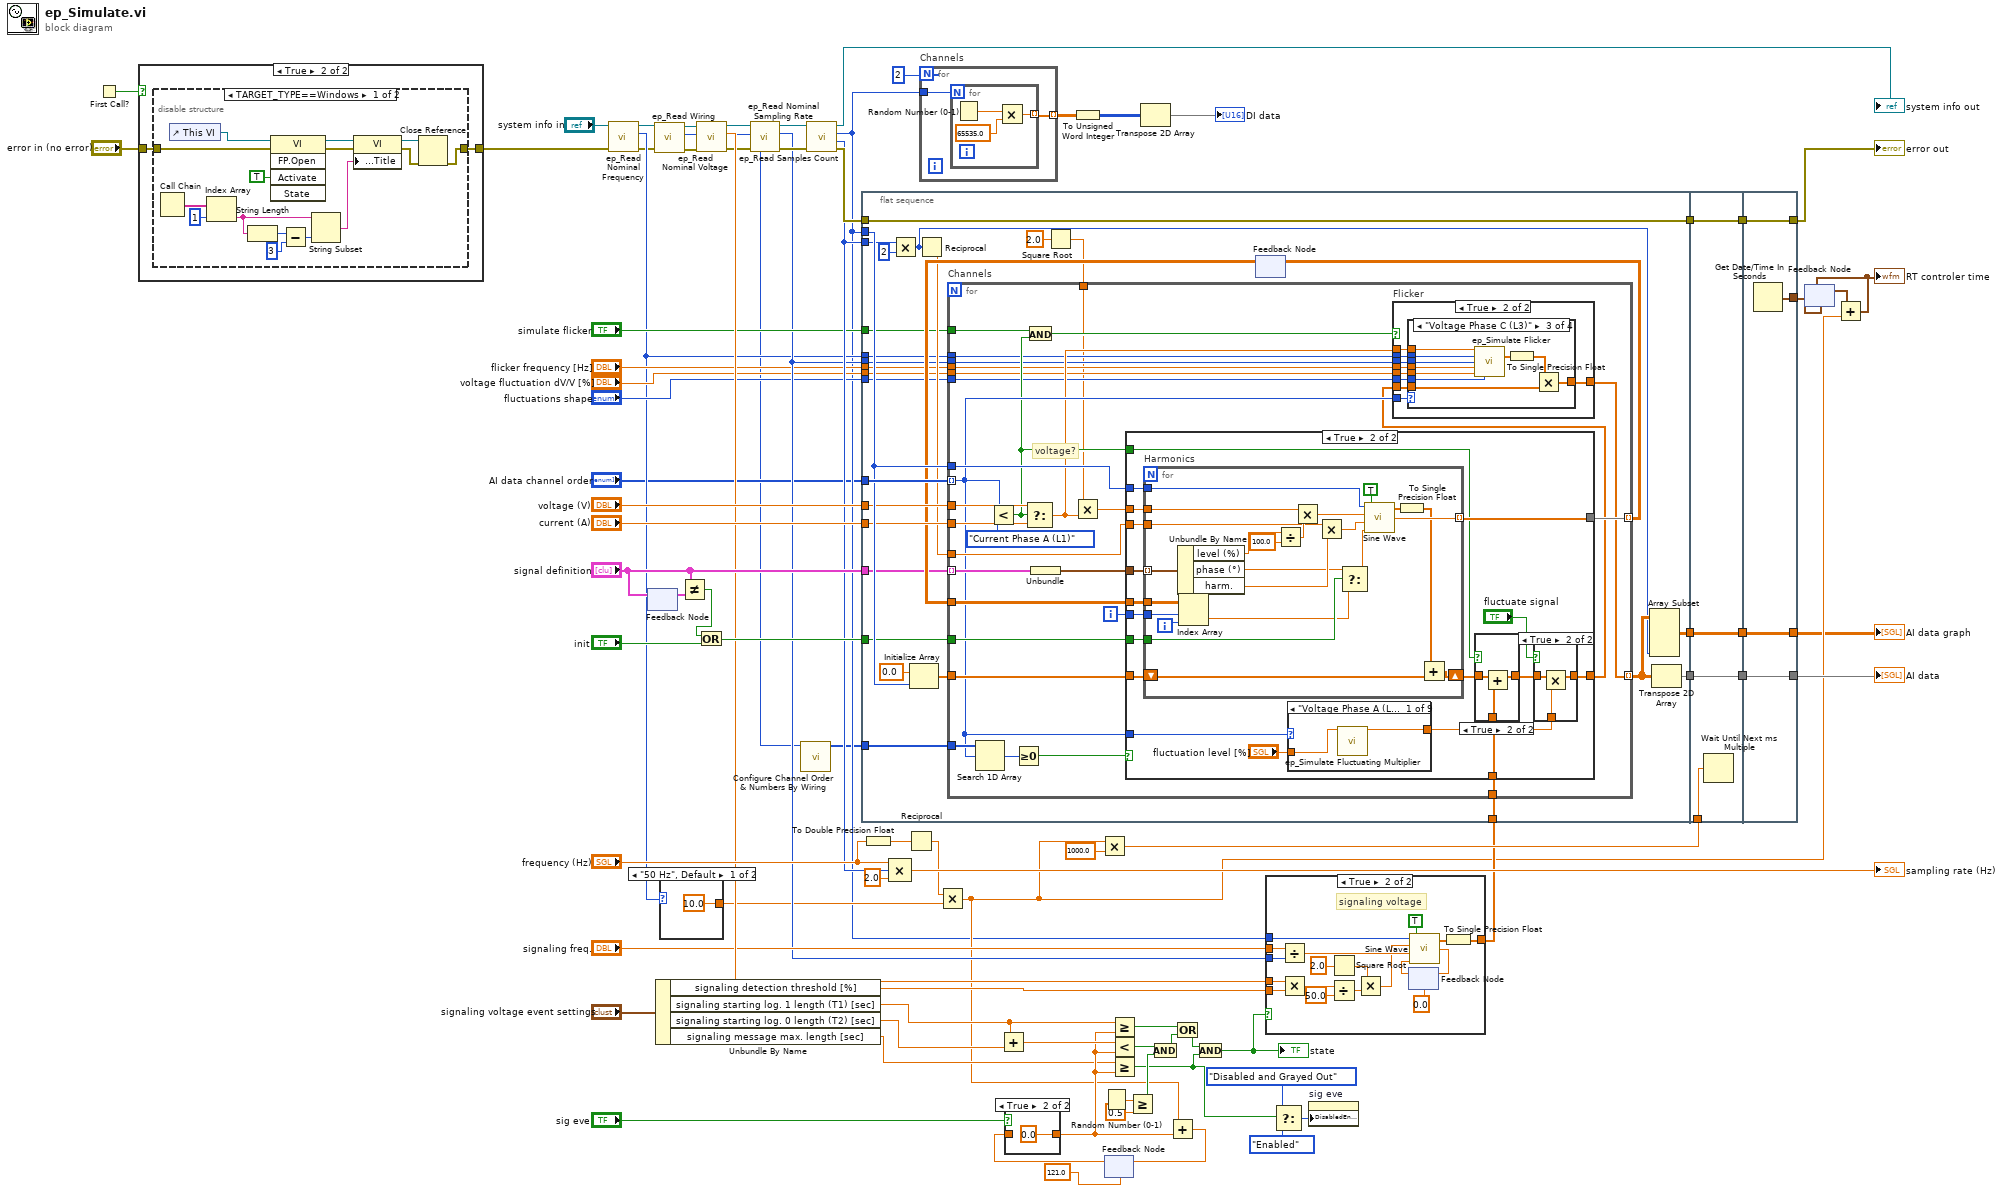
[diagram p0: block diagram]
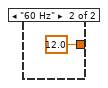
[diagram p4: hidden frame]
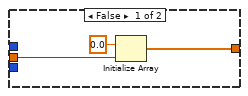
[diagram p6: hidden frame]
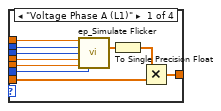
[diagram p8: hidden frame]
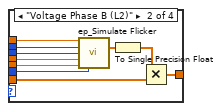
[diagram p9: hidden frame]
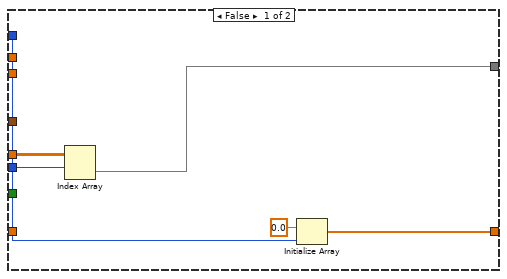
[diagram p11: hidden frame]
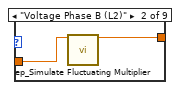
[diagram p12: hidden frame]
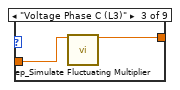
[diagram p13: hidden frame]
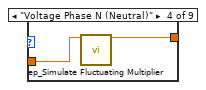
[diagram p14: hidden frame]
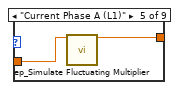
[diagram p15: hidden frame]
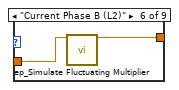
[diagram p16: hidden frame]
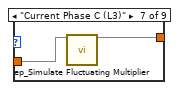
[diagram p17: hidden frame]
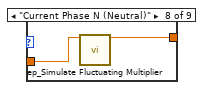
[diagram p18: hidden frame]
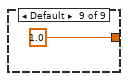
[diagram p19: hidden frame]
diagram:
  n1 = First Call?() -> (First Call?: T/F=w8:bool)
  n2 = case shown="True" w8 {
    tunnel: "error in (no error)" -> [w84 w86]
    tunnel: [w84 w85] -> w9
    frame False {
    }
    frame True {
      n3 = disable-structure shown="TARGET_TYPE==Windows" {
        disable-tunnel: w86 -> [w100 w102]
        disable-tunnel: [w87 w102] -> w85
        frame condition #0 (active) {
          n4 = Call Chain() -> (call chain=w98:string[])
          n5 = control-ref of="This VI"() -> (w99:refnum<vi>)
          n6 = Index Array(array=w98, index=1) -> (element=w94:string)
          n7 = String Length(string=w94) -> (length=w93:i32)
          n8 = invoke class="VI" method="FP.Open"(reference=w99, error in=w100, "Activate"=TRUE ("Activate?")) -> (reference out=w96:refnum<vi>, error out=w95:errorcluster)  [unwired: 2 in, 3 out]
          n9 = Subtract(x=w93, y=3) -> (x-y=w92:i32)
          n10 = String Subset(string=w94, length (rest)=w92) -> (substring=w90:string)  [unwired: 1 in]
          n11 = property class="VI"(reference=w96, error in=w95, "Front Panel.Title"=w90) -> (reference out=w89:refnum<vi>, error out=w88:errorcluster)
          n12 = Close Reference(reference=w89, error in (no error)=w88) -> (error out=w87:errorcluster)
        }
        frame condition #1 {
        }
      }
    }
  }
  n13 = call <vilib>:"ep_Read Nominal Frequency.vi"("error in (no error)"=w9, "system info in"="system info in") -> ("error out"=w5:errorcluster, "nominal frequency"=w20:enum16{"50 Hz", "60 Hz"}, "system info out"=w6:refnum<class "EP System Info.lvclass">)  [unwired: 6 in, 1 out]
  n14 = feedback-in #1("signal definition") -> ()
  n15 = feedback #1() -> (w67:T2)  [unwired: 1 in]
  n16 = call <vilib>:"ep_Read Wiring.vi"("error in (no error)"=w5, "system info in"=w6) -> ("error out"=w3:errorcluster, "wiring"=w2:T5, "system info out"=w4:refnum<class "EP System Info.lvclass">)  [unwired: 6 in, 1 out]
  n17 = Unbundle By Name("signaling voltage event settings") -> ("signaling detection threshold [%]"=w56:dbl, "signaling starting log. 1 length (T1) [sec]"=w55:dbl, "signaling starting log. 0 length (T2) [sec]"=w54:dbl, "signaling message max. length [sec]"=w40:dbl)
  n18 = case shown="\"50 Hz\", Default" w20 {
    tunnel: [10.0 ("y") 12.0 ("y")] -> w19
    frame "50 Hz", Default {
    }
    frame "60 Hz" {
    }
  }
  n19 = Not Equal?(x="signal definition", y=w67) -> (x != y?=w66:bool)
  n20 = call <vilib>:"ep_Read Nominal Voltage.vi"("error in (no error)"=w3, "system info in"=w4) -> ("error out"=w60:errorcluster, "nominal voltage [V]"=w65:dbl, "system info out"=w62:refnum<class "EP System Info.lvclass">)  [unwired: 7 in]
  n21 = Or(x=w66, y="init") -> (x .or. y?=w70:bool)
  n22 = call <vilib>:"ep_Read Nominal Sampling Rate.vi"("error in (no error)"=w60, "system info in"=w62) -> ("error out"=w59:errorcluster, "nominal sampling rate (Hz)"=w32:u16, "system info out"=w61:refnum<class "EP System Info.lvclass">)  [unwired: 7 in]
  n23 = call <vilib>:"Configure Channel Order & Numbers By Wiring.vi"("wiring"=w2) -> ("AI data channel order"=w1:T3[])  [unwired: 6 in, 4 out]
  n24 = call <vilib>:"ep_Read Samples Count.vi"("error in (no error)"=w59, "system info in"=w61) -> ("error out"=w83:errorcluster, "half-cycle (samples)"=w63:i32, "basic calc. interval (samples)"=w11:i32, "system info out"=→"system info out":refnum<class "EP System Info.lvclass">)  [unwired: 5 in, 1 out]
  n25 = flat-sequence {
    tunnel: w83 -> [w132]
    tunnel: [w132] -> w80
    tunnel: w11 -> [w129]
    tunnel: [w110] -> w78
    tunnel: "AI data channel order" -> [w131]
    tunnel: "voltage (V)" -> [w127]
    tunnel: "current (A)" -> [w126]
    tunnel: "signal definition" -> [w122]
    tunnel: w70 -> [w123]
    tunnel: w63 -> [w121]
    tunnel: w1 -> [w118]
    tunnel: w58 -> [w117]
    tunnel: "simulate flicker" -> [w116]
    tunnel: w20 -> [w115]
    tunnel: w32 -> [w114]
    tunnel: "flicker frequency [Hz]" -> [w113]
    tunnel: "voltage fluctuation dV/V [%]" -> [w112]
    tunnel: "fluctuations shape" -> [w111]
    tunnel: [w107] -> w26
    tunnel: w80 -> [w279]
    tunnel: [w279] -> w79
    tunnel: w78 -> [w278]
    tunnel: [w278] -> w77
    tunnel: w74 -> [w277]
    tunnel: [w276] -> w27
    tunnel: w26 -> [w276]
    tunnel: [w283] -> w82
    tunnel: w79 -> [w283]
    tunnel: [w280] -> w23
    tunnel: [w282] -> w28
    tunnel: w77 -> [w282]
    tunnel: [w281] -> w16
    tunnel: w27 -> [w281]
    frame #0 {
      n26 = Multiply(x=w121, y=2) -> (x*y=w105:i32)
      n27 = Initialize Array(sgl 0.0, w129) -> (w128:sgl[])
      n28 = Reciprocal(x=w105) -> (1/x=w119:dbl)
      n29 = Square Root(x=2.0) -> (sqrt(x)=w108:dbl)
      n30 = feedback #2() -> (w124:dbl[][])  [unwired: 1 in]
      n31 = for "Channels" {
        tunnel: w131 -> [w146] mode=indexing
        tunnel: w129 -> [w162]
        tunnel: w128 -> [w161]
        tunnel: [w160] -> w125 mode=indexing
        tunnel: [w136] -> w106 mode=indexing
        tunnel: w127 -> [w158]
        tunnel: w126 -> [w157]
        tunnel: w122 -> [w155] mode=indexing
        tunnel: w119 -> [w154]
        tunnel: w124 -> [w153]
        tunnel: w123 -> [w152]
        tunnel: w118 -> [w150]
        tunnel: w117 -> [w147]
        tunnel: w116 -> [w145]
        tunnel: w115 -> [w141]
        tunnel: w114 -> [w140]
        tunnel: w113 -> [w139]
        tunnel: w112 -> [w138]
        tunnel: w111 -> [w137]
        tunnel: w108 -> [w134]
        i -> [w151]
        # "voltage?"
        n32 = Search 1D Array(1D array=w150, element=w146) -> (index of element=w149:i32)  [unwired: 1 in]
        n33 = Less?(x=w146, y=ep_AI_Data_Channel."Current Phase A (L1)") -> (x < y?=w144:bool)
        n34 = Greater Or Equal To 0?(x=w149) -> (x >= 0?=w148:bool)
        n35 = Select(t=w158, s=w144, f=w157) -> (s? t:f=w142:dbl)
        n36 = And(x=w145, y=w144) -> (x .and. y?=w143:bool)
        n37 = Unbundle(w155) -> ("Array"=w133:T6)
        n38 = Multiply(x=w134, y=w142) -> (x*y=w156:dbl)
        n39 = case shown="True" w148 {
          tunnel: w162 -> [w206 w227]
          tunnel: w161 -> [_ w226]
          tunnel: [w207 w225] -> w160
          tunnel: [w204 w213] -> w135
          tunnel: w156 -> [_ w224]
          tunnel: w133 -> [_ w223]
          tunnel: w154 -> [_ w222]
          tunnel: w153 -> [w208 w221]
          tunnel: w152 -> [_ w220]
          tunnel: w151 -> [w209 w216]
          tunnel: w144 -> [_ w218]
          tunnel: w147 -> [_ w217]
          tunnel: w146 -> [_ w210]
          frame False {
            n40 = Index Array(array=w208, index (row)=w209) -> (element=w207:dbl[])  [unwired: 1 in]
            n41 = Initialize Array(sgl 0.0 ("element"), w206) -> (w204:sgl[])
          }
          frame True {
            n42 = for "Harmonics" {
              tunnel: w227 -> [w270]
              shift-right: [w253] -> w219
              shift-left: w226 -> [w274]
              tunnel: [w272] -> w225 mode=indexing
              tunnel: w224 -> [w265]
              tunnel: w223 -> [w269] mode=indexing
              tunnel: w222 -> [w262]
              tunnel: w221 -> [w255]
              tunnel: w220 -> [w259]
              tunnel: w216 -> [w257]
              i -> [w256]
              n43 = Unbundle By Name(w269) -> ("level (%)"=w268:dbl, "phase (°)"=w260:dbl, "harm."=w263:dbl)
              n44 = Index Array(array=w255, index (row)=w257, index (col)=w256) -> (element=w254:dbl)
              n45 = Divide(x=w268, y=100.0) -> (x/y=w266:dbl)
              n46 = Multiply(x=w265, y=w266) -> (x*y=w264:dbl)
              n47 = Multiply(x=w262, y=w263) -> (x*y=w261:dbl)
              n48 = Select(t=w260, s=w259, f=w254) -> (s? t:f=w258:dbl)
              n49 = call <vilib>:"Sine Wave.vi"("samples"=w270, "amplitude"=w264, "frequency"=w261, "phase in"=w258, "reset phase"=TRUE) -> ("sine wave"=w273:dbl[], "phase out"=w272:dbl)  [unwired: 1 out]
              n50 = To Single Precision Float(number=w273) -> (single precision float=w271:sgl[])
              n51 = Add(x=w271, y=w274) -> (x+y=w253:sgl[])
            }
            n52 = case shown="\"Voltage Phase A (L1)\"" w210 {
              tunnel: [w229 w231 w233 w235 w237 w239 w241 w243 sgl 1.0 ("multiplier")] -> w215
              tunnel: "fluctuation level [%]" -> [w228 w230 w232 w234 w236 w238 w240 w242 _]
              frame "Voltage Phase A (L1)" {
                n53 = call <vilib>:"ep_Simulate Fluctuating Multiplier.vi"("fluctuation level [%]"=w228) -> ("multiplier"=w229:sgl)  [unwired: 14 in]
              }
              frame "Voltage Phase B (L2)" {
                n54 = call <vilib>:"ep_Simulate Fluctuating Multiplier.vi"("fluctuation level [%]"=w230) -> ("multiplier"=w231:sgl)  [unwired: 14 in]
              }
              frame "Voltage Phase C (L3)" {
                n55 = call <vilib>:"ep_Simulate Fluctuating Multiplier.vi"("fluctuation level [%]"=w232) -> ("multiplier"=w233:sgl)  [unwired: 14 in]
              }
              frame "Voltage Phase N (Neutral)" {
                n56 = call <vilib>:"ep_Simulate Fluctuating Multiplier.vi"("fluctuation level [%]"=w234) -> ("multiplier"=w235:sgl)  [unwired: 14 in]
              }
              frame "Current Phase A (L1)" {
                n57 = call <vilib>:"ep_Simulate Fluctuating Multiplier.vi"("fluctuation level [%]"=w236) -> ("multiplier"=w237:sgl)  [unwired: 14 in]
              }
              frame "Current Phase B (L2)" {
                n58 = call <vilib>:"ep_Simulate Fluctuating Multiplier.vi"("fluctuation level [%]"=w238) -> ("multiplier"=w239:sgl)  [unwired: 14 in]
              }
              frame "Current Phase C (L3)" {
                n59 = call <vilib>:"ep_Simulate Fluctuating Multiplier.vi"("fluctuation level [%]"=w240) -> ("multiplier"=w241:sgl)  [unwired: 14 in]
              }
              frame "Current Phase N (Neutral)" {
                n60 = call <vilib>:"ep_Simulate Fluctuating Multiplier.vi"("fluctuation level [%]"=w242) -> ("multiplier"=w243:sgl)  [unwired: 14 in]
              }
              frame Default {
              }
            }
            n61 = case shown="True" w218 {
              tunnel: w219 -> [w249 w252]
              tunnel: [w249 w251] -> w214
              tunnel: w217 -> [_ w250]
              frame False {
              }
              frame True {
                n62 = Add(x=w252, y=w250) -> (x+y=w251:sgl[])
              }
            }
            n63 = case shown="True" "fluctuate signal" {
              tunnel: w214 -> [w245 w248]
              tunnel: [w245 w247] -> w213
              tunnel: w215 -> [_ w246]
              frame False {
              }
              frame True {
                n64 = Multiply(x=w248, y=w246) -> (x*y=w247:sgl[])
              }
            }
          }
        }
        n65 = case "Flicker" shown="True" w143 {
          tunnel: w146 -> [_ w172]
          tunnel: w135 -> [w163 w171]
          tunnel: [w163 w170] -> w136
          tunnel: w142 -> [_ w169]
          tunnel: w141 -> [_ w168]
          tunnel: w140 -> [_ w167]
          tunnel: w139 -> [_ w166]
          tunnel: w138 -> [_ w165]
          tunnel: w137 -> [_ w164]
          frame False {
          }
          frame True {
            n66 = case shown="\"Voltage Phase C (L3)\"" w172 {
              tunnel: w171 -> [w181 w191 w201 w203]
              tunnel: [w180 w190 w200 w203] -> w170
              tunnel: w169 -> [w179 w189 w199 _]
              tunnel: w168 -> [w178 w188 w198 _]
              tunnel: w167 -> [w177 w187 w197 _]
              tunnel: w166 -> [w176 w186 w196 _]
              tunnel: w165 -> [w175 w185 w195 _]
              tunnel: w164 -> [w174 w184 w194 _]
              frame "Voltage Phase A (L1)" {
                n67 = call <vilib>:"ep_Simulate Flicker.vi"("amplitude RMS [V]"=w179, "nominal frequency"=w178, "nominal sampling rate (Hz)"=w177, "flicker frequency [Hz]"=w176, "voltage fluctuation dV/V [%]"=w175, "fluctuations shape"=w174) -> ("data multiplier"=w182:dbl[])  [unwired: 8 in, 1 out]
                n68 = To Single Precision Float(number=w182) -> (single precision float=w173:sgl[])
                n69 = Multiply(x=w173, y=w181) -> (x*y=w180:sgl[])
              }
              frame "Voltage Phase B (L2)" {
                n70 = call <vilib>:"ep_Simulate Flicker.vi"("amplitude RMS [V]"=w189, "nominal frequency"=w188, "nominal sampling rate (Hz)"=w187, "flicker frequency [Hz]"=w186, "voltage fluctuation dV/V [%]"=w185, "fluctuations shape"=w184) -> ("data multiplier"=w192:dbl[])  [unwired: 8 in, 1 out]
                n71 = To Single Precision Float(number=w192) -> (single precision float=w183:sgl[])
                n72 = Multiply(x=w183, y=w191) -> (x*y=w190:sgl[])
              }
              frame "Voltage Phase C (L3)" {
                n73 = call <vilib>:"ep_Simulate Flicker.vi"("amplitude RMS [V]"=w199, "nominal frequency"=w198, "nominal sampling rate (Hz)"=w197, "flicker frequency [Hz]"=w196, "voltage fluctuation dV/V [%]"=w195, "fluctuations shape"=w194) -> ("data multiplier"=w202:dbl[])  [unwired: 8 in, 1 out]
                n74 = To Single Precision Float(number=w202) -> (single precision float=w193:sgl[])
                n75 = Multiply(x=w193, y=w201) -> (x*y=w200:sgl[])
              }
              frame Default {
              }
            }
          }
        }
      }
      n76 = feedback-in #2(w125) -> ()
      n77 = Array Subset(array=w106, length (col)=w105) -> (w107:sgl[][])  [unwired: 3 in]
      n78 = Transpose 2D Array(2D array=w106) -> (transposed array=w110:sgl[][])
    }
    frame #1 {
      n79 = Wait Until Next ms Multiple(millisecond multiple=w277) -> ()  [unwired: 1 out]
    }
    frame #2 {
      n80 = Get Date/Time In Seconds() -> (seconds since 1Jan1904=w280:timestamp)
    }
  }
  n81 = To Double Precision Float(number="frequency (Hz)") -> (double precision float=w25:dbl)
  n82 = Compound Arithmetic op=MULTIPLY("frequency (Hz)", w63, sgl 2.0 ("value")) -> (→"sampling rate (Hz)":sgl)
  n83 = Reciprocal(x=w25) -> (1/x=w22:dbl)
  n84 = for "Channels" {
    N: 2 -> [_]
    tunnel: w11 -> [w285]
    tunnel: [w284] -> w13 mode=indexing
    n85 = for {
      N: w285 -> [_]
      tunnel: [w288] -> w284 mode=indexing
      n86 = Random Number (0-1)() -> (number: 0 to 1=w287:dbl)
      n87 = Multiply(x=w287, y=65535.0) -> (x*y=w288:dbl)
    }
  }
  n88 = Multiply(x=w22, y=w19) -> (x*y=w18:dbl)
  n89 = Add(x=w55, y=w54) -> (x+y=w50:dbl)
  n90 = To Unsigned Word Integer(number=w13) -> (unsigned 16bit integer=w15:u16[][])
  n91 = Multiply(x=w18, y=1000.0) -> (x*y=w74:dbl)
  n92 = Random Number (0-1)() -> (number: 0 to 1=w45:dbl)
  n93 = feedback #3(121.0) -> (w41:dbl)
  n94 = case shown="True" "sig eve" {
    tunnel: [w289 0.0] -> w47
    tunnel: w41 -> [w289 _]
    frame False {
    }
    frame True {
    }
  }
  n95 = Greater Or Equal?(x=w55, y=w47) -> (x >= y?=w51:bool)
  n96 = Less?(x=w50, y=w47) -> (x < y?=w48:bool)
  n97 = Greater Or Equal?(x=w40, y=w47) -> (x >= y?=w35:bool)
  n98 = Greater Or Equal?(x=w45, y=0.5) -> (x >= y?=w43:bool)
  n99 = Transpose 2D Array(2D array=w15) -> (transposed array=→"DI data":u16[][])
  n100 = And(x=w48, y=w43) -> (x .and. y?=w49:bool)
  n101 = Add(x=w18, y=w47) -> (x+y=w42:dbl)
  n102 = feedback-in #3(w42) -> ()
  n103 = Or(x=w51, y=w49) -> (x .or. y?=w46:bool)
  n104 = And(x=w46, y=w35) -> (x .and. y?=w52:bool)
  "state" <- w52
  n105 = case shown="True" w52 {
    tunnel: w11 -> [w292 w309]
    tunnel: [w291 w308] -> w58
    tunnel: w65 -> [_ w306]
    tunnel: "signaling freq." -> [_ w302]
    tunnel: w32 -> [_ w303]
    tunnel: w56 -> [_ w294]
    frame False {
      n106 = Initialize Array(sgl 0.0 ("element"), w292) -> (w291:sgl[])
    }
    frame True {
      # "signaling voltage"
      n107 = Divide(x=w302, y=w303) -> (x/y=w300:dbl)
      n108 = Multiply(x=w306, y=w294) -> (x*y=w305:dbl)
      n109 = Square Root(x=2.0) -> (sqrt(x)=w298:dbl)
      n110 = Divide(x=w305, y=50.0) -> (x/y=w296:dbl)
      n111 = Multiply(x=w298, y=w296) -> (x*y=w297:dbl)
      n112 = feedback #4(0.0 ("phase out")) -> (w295:dbl)
      n113 = call <vilib>:"Sine Wave.vi"("samples"=w309, "amplitude"=w297, "frequency"=w300, "phase in"=w295, "reset phase"=TRUE) -> ("sine wave"=w311:dbl[], "phase out"=w307:dbl)  [unwired: 1 out]
      n114 = feedback-in #4(w307) -> ()
      n115 = To Single Precision Float(number=w311) -> (single precision float=w308:sgl[])
    }
  }
  n116 = Select(t=T4."Disabled and Grayed Out" ("Disabled"), s=w35, f=T4."Enabled" ("Disabled")) -> (s? t:f=w36:T4)
  n117 = property on="sig eve" class="Bool"("DisabledEnum"=w36) -> ()  [unwired: 2 in, 2 out]
  n118 = feedback #5(w23) -> (w24:timestamp)
  n119 = Add(x=w24, y=w18) -> (x+y=w21:timestamp)
  "RT controler time" <- w21
  n120 = feedback-in #5(w21) -> ()
  "error out" <- w82
  "AI data" <- w28
  "AI data graph" <- w16
